vi "Ardunio_Terminal.vi"() -> ()   [LabVIEW 2012]
uses:
  <userlib>/botspeak/VIs/Direct/BotSpeak_Control.ctl
panel:
  out "Version":string
  in  "stop":bool
  out "Analog":dbl[](array[numeric])
  in  "DIO states":bool[](array[boolean])
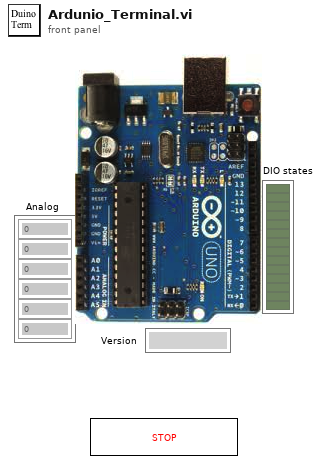
[diagram p1: front panel]
types:
  T1 = typedef "BotSpeak_Control.ctl" = cluster{"Address":string, "Reply EOF":string, "Hardware":string, "Retries":i8, "Timeout":i32, "Open?":bool}
  T2 = enum8{"Enabled", "Disabled", "Disabled and Grayed Out"}
  T3 = typedef "URAPI_Control.ctl" = cluster{"Script":string, "Whiles":u8[], "Ifs":u8[], "Supress Err":bool, "Errors":string}
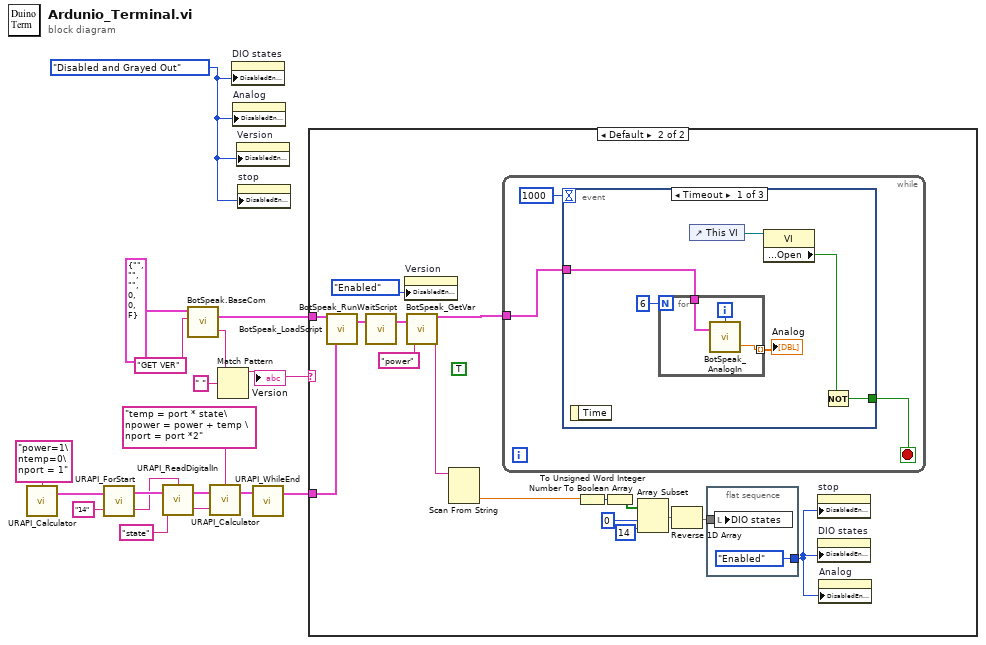
[diagram p0: block diagram]
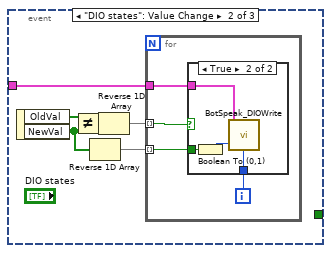
[diagram p3: hidden frame]
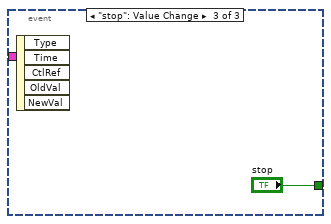
[diagram p5: hidden frame]
diagram:
  w4 = T2."Disabled and Grayed Out" ("Disabled")
  n1 = call <userlib>:"URAPI_Calculator.vi"("Formula"="power=1\ntemp=0\nport = 1") -> ("URAPI Script"=w11:T3)  [unwired: 3 in, 1 out]
  n2 = call <userlib>:"URAPI_ForStart.vi"("Iterations"="14", "URAPI Script"=w11) -> ("variable"=w16:string, "URAPI Script Out"=w17:T3)  [unwired: 2 in]
  n3 = call <userlib>:"URAPI_ReadDigitalIn.vi"("Variable In"="state", "URAPI Script"=w17, "Channel"=w16) -> ("Variable Out"=w14:string, "URAPI Script"=w15:T3)  [unwired: 1 in]
  n4 = call <userlib>:"BotSpeak.BaseCom.vi"("command"="GET VER", "Bot Settings in"=T1 {"Address"="", "Reply EOF"="", "Hardware"="", "Retries"=0, "Timeout"=0, "Open?"=FALSE} ("Bot Settings")) -> ("response"=w3:string, "Bot Settings out"=w6:T1)  [unwired: 3 in]
  n5 = call <userlib>:"URAPI_Calculator.vi"("X"=w14, "URAPI Script"=w15, "Formula"="temp = port * state\npower = power + temp \nport = port *2") -> ("URAPI Script"=w13:T3)  [unwired: 1 in, 1 out]
  n6 = Match Pattern(string=w3, regular expression=" ") -> (before substring=w1:string)  [unwired: 1 in, 3 out]
  "Version" <- w1
  n7 = property on="DIO states" class="Arr (strict)"("DisabledEnum"=w4) -> ()  [unwired: 2 in, 2 out]
  n8 = property on="Analog" class="Arr (strict)"("DisabledEnum"=w4) -> ()  [unwired: 2 in, 2 out]
  n9 = property on="Version" class="Str"("DisabledEnum"=w4) -> ()  [unwired: 2 in, 2 out]
  n10 = property on="stop" class="Bool"("DisabledEnum"=w4) -> ()  [unwired: 2 in, 2 out]
  n11 = call <userlib>:"URAPI_WhileEnd.vi"("URAPI Script"=w13) -> ("URAPI Script Out"=w8:T3)  [unwired: 4 in]
  n12 = case shown="Default" w1 {
    tunnel: w8 -> [_ w26]
    tunnel: w6 -> [_ w25]
    frame "" {
    }
    frame Default {
      (unwired) TRUE
      n13 = call <userlib>:"BotSpeak_LoadScript.vi"("URAPI Script"=w26, "Bot Settings"=w25) -> ("Bot Settings"=w22:T1)  [unwired: 1 out]
      n14 = call <userlib>:"BotSpeak_RunWaitScript.vi"("Bot Settings"=w22) -> ("Bot Settings"=w21:T1)  [unwired: 1 in, 1 out]
      n15 = property on="Version" class="Str"("DisabledEnum"=T2."Enabled" ("Disabled")) -> ()  [unwired: 2 in, 2 out]
      n16 = call <userlib>:"BotSpeak_GetVar.vi"("Variable In"="power", "Bot Settings"=w21) -> ("response"=w24:string, "Bot Settings out"=w28:T1)
      n17 = Scan From String(input string=w24) -> (output 1=w27:dbl)  [unwired: 4 in, 3 out]
      n18 = while {
        tunnel: w28 -> [w37]
        stop <- w38 stop-if-true
        n19 = event shown="[0] Timeout" {
          selector: _ -> [_ _ _]
          dyn-events: _ -> [_ _ _]
          timeout: 1000 -> [_ _ _]
          tunnel: w37 -> [w43 w49 _]
          tunnel: [w40 _ "stop"] -> w38
          event Timeout {
            n20 = event-data() -> ()  [unwired: 1 in, 1 out]
            n21 = for {
              N: 6 -> [_]
              tunnel: [w46] -> w44 mode=indexing
              tunnel: w43 -> [w48]
              i -> [w47]
              n22 = call <userlib>:"BotSpeak_AnalogIn.vi"("Bot Settings"=w48, "A/D Channel"=w47) -> ("voltage"=w46:dbl)  [unwired: 1 in, 1 out]
            }
            "Analog" <- w44
            n23 = control-ref of="This VI"() -> (w42:refnum<vi>)
            n24 = property class="VI"(reference=w42) -> ("Front Panel.Open"=w41:bool)  [unwired: 1 in, 2 out]
            n25 = Not(x=w41) -> (.not. x?=w40:bool)
          }
          event "DIO states": Value Change {
            n26 = event-data() -> ("OldVal"=w54:bool[], "NewVal"=w52:bool[])  [unwired: 1 in]
            n27 = Not Equal?(x=w54, y=w52) -> (x != y?=w53:bool[])
            n28 = Reverse 1D Array(array=w52) -> (reversed array=w50:bool[])
            n29 = Reverse 1D Array(array=w53) -> (reversed array=w51:bool[])
            n30 = for {
              tunnel: w51 -> [w58] mode=indexing
              tunnel: w50 -> [w55] mode=indexing
              tunnel: w49 -> [w56]
              i -> [w57]
              n31 = case shown="True" w58 {
                tunnel: w57 -> [_ w59]
                tunnel: w55 -> [_ w62]
                tunnel: w56 -> [_ w61]
                frame False {
                }
                frame True {
                  n32 = Boolean To (0,1)(Boolean=w62) -> (0, 1=w60:i16)
                  n33 = call <userlib>:"BotSpeak_DIOWrite.vi"("State"=w60, "Bot Settings"=w61, "DIO Line"=w59) -> ()  [unwired: 1 in, 1 out]
                }
              }
            }
          }
          event "stop": Value Change {
            n34 = event-data() -> ()  [unwired: 1 in, 5 out]
          }
        }
      }
      n35 = To Unsigned Word Integer(number=w27) -> (unsigned 16bit integer=w33:u16)
      n36 = Number To Boolean Array(number=w33) -> (Boolean array=w31:bool[])
      n37 = Array Subset(array=w31, index=0, length=14) -> (w32:bool[])
      n38 = Reverse 1D Array(array=w32) -> (reversed array=w34:bool[])
      n39 = flat-sequence {
        tunnel: [T2."Enabled" ("Disabled")] -> w19
        tunnel: w34 -> [w35]
        frame #0 {
          n40 = local write "DIO states"(w35) -> ()
        }
      }
      n41 = property on="stop" class="Bool"("DisabledEnum"=w19) -> ()  [unwired: 2 in, 2 out]
      n42 = property on="DIO states" class="Arr (strict)"("DisabledEnum"=w19) -> ()  [unwired: 2 in, 2 out]
      n43 = property on="Analog" class="Arr (strict)"("DisabledEnum"=w19) -> ()  [unwired: 2 in, 2 out]
    }
  }
